vi "New I2C Device.vi"(7 "I2C Slave Address":u8 format="%.0x", 8 "error in (no error)":errorcluster, 10 "I2C Channel":u8, 11 "object in":T1) -> (0 "error out":errorcluster, 3 "mainI2CDevice out":refnum<class "mainI2CDevice.lvclass">)   [LabVIEW 2020, in "RPI.lvlib" / "mainI2CDevice.lvclass"]
doc: "Initialize the mainI2CDevice object and open the specified I2C channel."
uses:
  mainI2CDevice.lvclass
  <vilib>/MakerHub/LINX/Private/Type Defs/LINX Ref.ctl
  <vilib>/MakerHub/LINX/Private/Type Defs/Platform.ctl
  <vilib>/MakerHub/LINX/Private/Type Defs/Interface.ctl
  <vilib>/MakerHub/LINX/Private/Device/Type Defs/LINX Device Config.ctl
  <vilib>/MakerHub/LINX/Private/Device/Type Defs/TCP Config.ctl
  <vilib>/MakerHub/LINX/Private/Device/Type Defs/Channels.ctl
  mainI2CDevice.lvclass/mainI2CDevice.ctl
  <vilib>/MakerHub/LINX/LMH-LINX.lvlib
  <vilib>/MakerHub/LINX/Private/Device/Device.lvlib
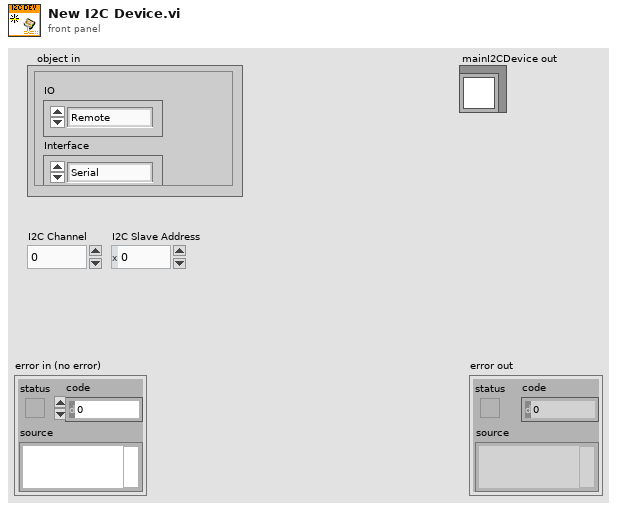
[diagram p1: front panel]
types:
  T1 = typedef "LMH-LINX.lvlib/LINX Ref.ctl" = cluster{"IO":T2, "Interface":T3, "LINX Device Config":T4}
  T2 = typedef "LMH-LINX.lvlib/Platform.ctl" = enum16{"Remote", "Local"}
  T3 = typedef "LMH-LINX.lvlib/Interface.ctl" = enum16{"Serial", "TCP"}
  T4 = typedef "LMH-LINX.lvlib/Device.lvlib/LINX Device Config.ctl" = cluster{"Interface":T3, "COM Port":refnum<visa-resource-name>, "TCP Configuration":T5, "Device Family":u8, "Device ID":u8, "Device Name":string, "TCP Ref":refnum<k5>, "Channels":T6}
  T5 = typedef "LMH-LINX.lvlib/Device.lvlib/TCP Config.ctl" = cluster{"IP Address":string, "Port":u16}
  T6 = typedef "LMH-LINX.lvlib/Channels.ctl" = cluster{"DI":u8[], "DO":u8[], "AI":u8[], "AO":u8[], "PWM":u8[], "QE":u8[], "UART":u8[], "I2C 2":u8[], "SPI":u8[], "CAN":u8[], "Servo":u8[], "AI Ref (V)":dbl, "AI Resolution (Bits)":u8, "AO Ref (V)":dbl, "AO Resolution (Bits)":u8}
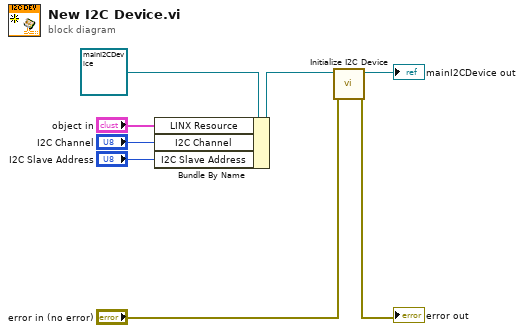
[diagram p0: block diagram]
diagram:
  n1 = Bundle By Name(cluster=refnum<class "mainI2CDevice.lvclass"> refnum ("object out"), "LINX Resource"="object in", "I2C Channel"="I2C Channel", "I2C Slave Address"="I2C Slave Address") -> (w6:refnum<class "mainI2CDevice.lvclass">)
  n2 = call "Initialize I2C Device.vi"("error in (no error)"="error in (no error)", "mainI2CDevice in"=w6) -> ("error out"=→"error out":errorcluster, "mainI2CDevice out"=→"mainI2CDevice out":refnum<class "mainI2CDevice.lvclass">)  [unwired: 8 in]
